vi "Worker Name and Path.vi"(10 "Variant":string, 11 "Worker":string) -> (0 "error out":errorcluster, 1 "Is Worker Variant":bool, 2 "lvlib Path":path, 3 "Display Name":string)   [LabVIEW 2020, in "FlexBlocks.lvlib"]
uses:
  FlexBlocks.lvlib
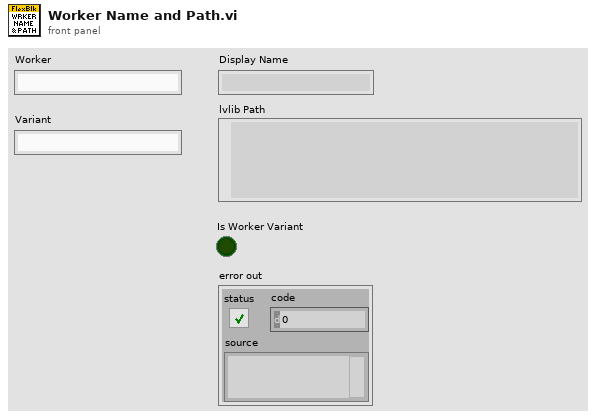
[diagram p1: front panel]
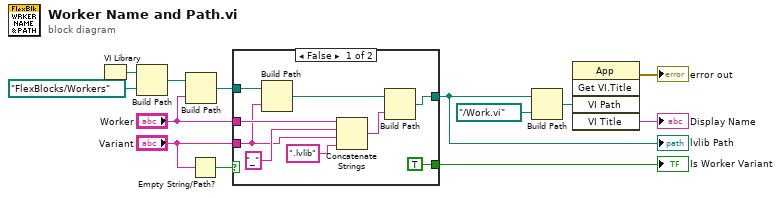
[diagram p0: block diagram]
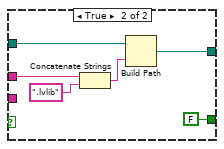
[diagram p2: hidden frame]
diagram:
  n1 = VI Library() -> (path=w13:path)
  n2 = Build Path(base path=w13, name or relative path=path "FlexBlocks/Workers") -> (appended path=w11:path)
  n3 = Build Path(base path=w11, name or relative path="Worker") -> (appended path=w7:path)
  n4 = Empty String/Path?(string/path="Variant") -> (empty?=w10:bool)
  n5 = case shown="False" w10 {
    tunnel: "Variant" -> [w19 _]
    tunnel: "Worker" -> [w22 w28]
    tunnel: w7 -> [w20 w26]
    tunnel: [w15 w24] -> w3
    tunnel: [TRUE FALSE] -> w4
    frame False {
      n6 = Build Path(base path=w20, name or relative path=w19) -> (appended path=w17:path)
      n7 = Concatenate Strings(w22, "_" ("string"), w19, ".lvlib" ("string")) -> (w16:string)
      n8 = Build Path(base path=w17, name or relative path=w16) -> (appended path=w15:path)
    }
    frame True {
      n9 = Concatenate Strings(w28, ".lvlib" ("string")) -> (w25:string)
      n10 = Build Path(base path=w26, name or relative path=w25) -> (appended path=w24:path)
    }
  }
  "lvlib Path" <- w3
  "Is Worker Variant" <- w4
  n11 = Build Path(base path=w3, name or relative path=path "../Work.vi") -> (appended path=w1:path)
  n12 = invoke class="App" method="Get VI.Title"("VI Path"=w1) -> (error out=→"error out":errorcluster, "VI Title"=→"Display Name":string)  [unwired: 4 in, 3 out]
